vi "global_variable_GAUGE_PANEL_ERROR.vi"() -> ()   [LabVIEW 2017]
panel:
  in  "GAUGE PANEL ERROR":bool
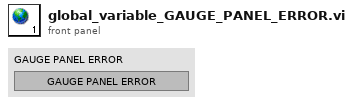
[diagram p1: front panel]
diagram:
